vi "IN-0-OpAmp3.vi"(5 "Rf(kW)":dbl(slide)=50.0 min=10.0 max=100.0 scale=10.0..100.0 scale format="%.1f", 6 "Vin":dbl=-1.25 format="%.2f", 7 "R1(kW)":dbl(slide)=20.0 min=1.0 max=50.0 scale=1.0..50.0 scale format="%.1f") -> (1 "Vout":dbl(knob)=5.0 min=-15.0 max=15.0 scale=-15.0..15.0 scale format="%.1f")   [LabVIEW 2010]
panel:
  out "Message Center 3":string
  out "Message Center2":string
  out "Message Center1":string
  in  "help":bool
  # "[Press Run]"
  # "-"
  # "+"
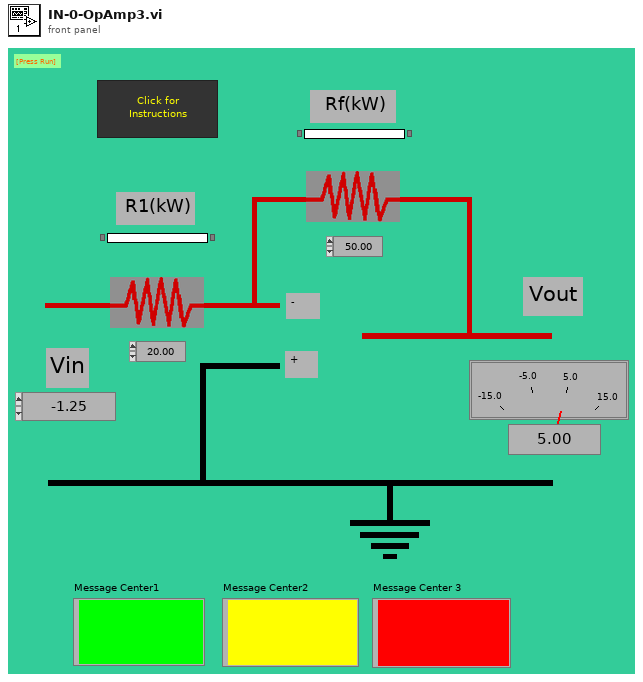
[diagram p1: front panel]
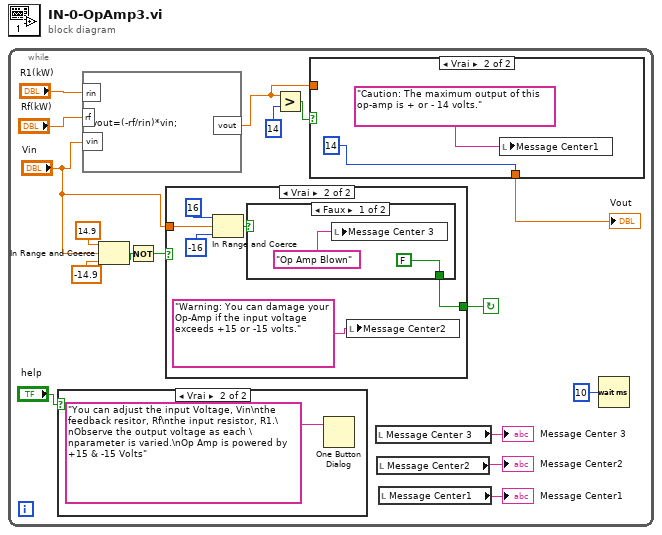
[diagram p0: block diagram]
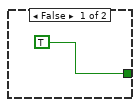
[diagram p3: hidden frame]
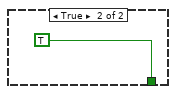
[diagram p4: hidden frame]
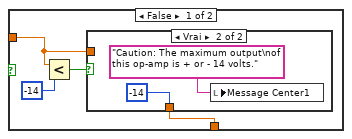
[diagram p5: hidden frame]
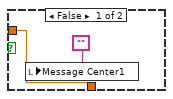
[diagram p6: hidden frame]
diagram:
  n1 = while {
    stop <- w11 continue-if-true
    n2 = case shown="Vrai" "help" {
      frame False {
      }
      frame True {
        n3 = One Button Dialog(message="You can adjust the input Voltage, Vin\nthe feedback resitor, Rf\nthe input resistor, R1.\nObserve the output voltage as each \nparameter is varied.\nOp Amp is powered by +15 & -15 Volts") -> ()  [unwired: 1 in, 1 out]
      }
    }
    n4 = formula code="vout=(-rf/rin)*vin;"("rin"="R1(kW)", "rf"="Rf(kW)", "vin"="Vin") -> ("vout"=w12:dbl)
    n5 = In Range and Coerce(upper limit=14.9, x="Vin", lower limit=-14.9) -> (In Range?=w2:bool)  [unwired: 1 out]
    n6 = Not(x=w2) -> (.not. x?=w1:bool)
    n7 = case shown="Vrai" w1 {
      tunnel: "Vin" -> [_ w22]
      tunnel: [TRUE w25] -> w11
      frame False {
      }
      frame True {
        n8 = In Range and Coerce(upper limit=16, x=w22, lower limit=-16) -> (In Range?=w21:bool)  [unwired: 1 out]
        n9 = case shown="Faux" w21 {
          tunnel: [FALSE TRUE] -> w25
          frame False {
            n10 = local write "Message Center 3"("Op Amp Blown" ("Message Center 3")) -> ()
          }
          frame True {
          }
        }
        n11 = local write "Message Center2"("Warning: You can damage your Op-Amp if the input voltage exceeds +15 or -15 volts.") -> ()
      }
    }
    n12 = Greater?(x=w12, y=14) -> (0:w14:bool)
    n13 = case shown="Vrai" w14 {
      tunnel: [w30 14] -> w13
      tunnel: w12 -> [w29 _]
      frame False {
        n14 = Less?(x=w29, y=-14) -> (x < y?=w31:bool)
        n15 = case shown="Vrai" w31 {
          tunnel: [w34 -14] -> w30
          tunnel: w29 -> [w34 _]
          frame False {
            n16 = local write "Message Center1"("") -> ()
          }
          frame True {
            n17 = local write "Message Center1"("Caution: The maximum output\nof this op-amp is + or - 14 volts.") -> ()
          }
        }
      }
      frame True {
        n18 = local write "Message Center1"("Caution: The maximum output of this op-amp is + or - 14 volts.") -> ()
      }
    }
    "Vout" <- w13
    n19 = local read "Message Center 3"() -> (→"Message Center 3":string)
    n20 = local read "Message Center2"() -> (→"Message Center2":string)
    n21 = local read "Message Center1"() -> (→"Message Center1":string)
    n22 = Wait (ms)(milliseconds to wait=u32 10) -> ()  [unwired: 1 out]
  }
